vi "SECoP_dataGetInfo.vi"(7 "Position":u32, 8 "error in (no error)":errorcluster, 10 "SECoP_dataPtr":T1 {"ptr64" format="%.0x"; "ptr32" format="%.0x"}, 11 "DLL path (in)":T3) -> (0 "error out":errorcluster, 1 "Name":string, 2 "Type":T2 items=["NONE"=0, "DOUBLE"=1, "INTEGER"=2, "BOOL"=3, "ENUM"=4, "SCALED"=5, "ARRAY"=10, "ARRAY_DOUBLE"=11, "ARRAY_INTEGER"=12, "ARRAY_BOOL"=13, "ARRAY_ENUM"=14, "ARRAY_SCALED"=15, "STRING"=20, "BLOB"=21, "JSON"=22, "STRUCT"=30, "TUPLE"=31, "COMMAND"=40], 3 "DLL path (out)":T3, 5 "Count":u32)   [LabVIEW 2023, in "SECoP.lvlib"]
doc: "Call <b>\"SECoP_dataGetInfo.vi\"</b> to access the numeric value (integer or scaled of SECoP_dataPtr).\n\n<b>DLL path</b> input and output of cluster from \"SECoP-Initialize.vi\"\n<b>SECoP_dataPtr</b> data to access\n<b>Position</b> zero based index points to a virtual flattened entry of the data type\n<b>Type</b> data type of selected element\n<b>Count</b> for array/struct/tuple a length or count of elements, for single type should be 1\n<b>Name</b> name of selected structure item or empty (no struct)"
uses:
  SECoP.lvlib
  SECoP-libraries.ctl
  SECoP-dataType.ctl
  SECoP-data.ctl
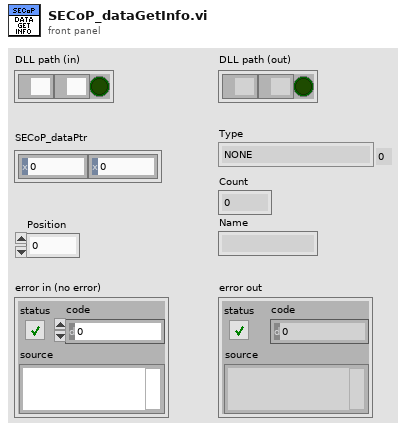
[diagram p1: front panel]
types:
  T1 = typedef "SECoP.lvlib/SECoP-data.ctl" = cluster{"ptr32":u32, "ptr64":u64}
  T2 = typedef "SECoP.lvlib/SECoP-dataType.ctl" = u32
  T3 = typedef "SECoP.lvlib/SECoP-libraries.ctl" = cluster{"serverDLL":path, "variantDLL":path, "cleanup_mode":bool}
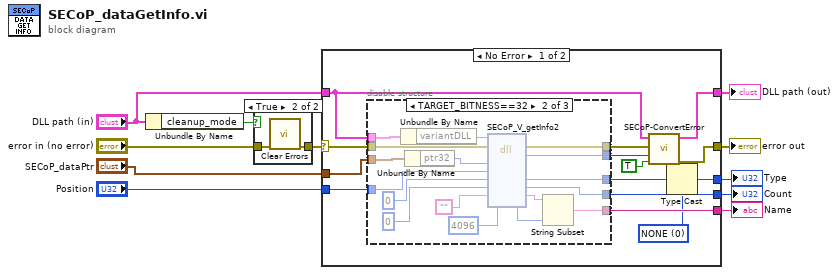
[diagram p0: block diagram]
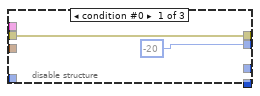
[diagram p3: hidden frame]
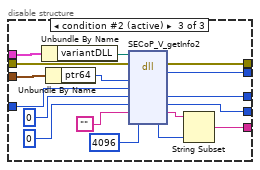
[diagram p4: hidden frame]
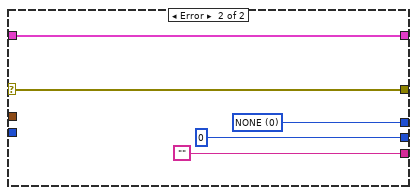
[diagram p5: hidden frame]
diagram:
  n1 = Unbundle By Name("DLL path (in)") -> ("cleanup_mode"=w8:bool)
  n2 = case shown="True" w8 {
    tunnel: "error in (no error)" -> [w12 w14]
    tunnel: [w12 w13] -> w6
    frame False {
    }
    frame True {
      n3 = call <vilib>:"Clear Errors.vi"("error in (no error)"=w14) -> ("error out"=w13:errorcluster)  [unwired: 5 in, 1 out]
    }
  }
  n4 = case shown="No Error" w6 {
    selector: w6 -> [w26 w68]
    tunnel: "DLL path (in)" -> [w18 w69]
    tunnel: [w27 w69] -> w10
    tunnel: [w28 w68] -> w9
    tunnel: "Position" -> [w23 _]
    tunnel: [w15 w65] -> w4
    tunnel: [w21 ""] -> w3
    tunnel: [w22 u32 0 ("Count")] -> w2
    tunnel: "SECoP_dataPtr" -> [w19 _]
    frame No Error {
      w16 = T2 0 items=["NONE"=0, "DOUBLE"=1, "INTEGER"=2, "BOOL"=3, "ENUM"=4, "SCALED"=5, "ARRAY"=10, "ARRAY_DOUBLE"=11, "ARRAY_INTEGER"=12, "ARRAY_BOOL"=13, "ARRAY_ENUM"=14, "ARRAY_SCALED"=15, "STRING"=20, "BLOB"=21, "JSON"=22, "STRUCT"=30, "TUPLE"=31, "COMMAND"=40] ("SECoP data type")
      n5 = disable-structure shown="TARGET_BITNESS==32" {
        disable-tunnel: w26 -> [w30 w47 w64]
        disable-tunnel: w18 -> [_ w46 w63]
        disable-tunnel: [w30 w45 w62] -> w25
        disable-tunnel: [-20 w44 w61] -> w24
        disable-tunnel: w23 -> [_ w43 w60]
        disable-tunnel: [_ w42 w59] -> w17
        disable-tunnel: [_ w40 w57] -> w22
        disable-tunnel: [_ w35 w52] -> w21
        disable-tunnel: w19 -> [_ w33 w51]
        frame condition #0 {
        }
        frame condition #1 {
          n6 = Unbundle By Name(w46) -> ("variantDLL"=w31:path)
          n7 = Unbundle By Name(w33) -> ("ptr32"=w32:u32)
          n8 = dll-call lib="Z:/Praktische_Aufgaben/SECoP-LabVIEW2015/32bit/SECoP32.dll" fn="SECoP_V_getInfo2"(path in=w31, error in=w47, "Data"=w32, "Position"=w43, "Type"=0, "Count"=u32 0, "Name"="", "name length"=4096) -> (error out=w45:errorcluster, "return type"=w44:i32, "Type"=w42:i32, "Count"=w40:u32, "Name"=w41:string, "name length"=w34:i32)  [unwired: 3 in, 1 out]
          n9 = String Subset(string=w41, length (rest)=w34) -> (substring=w35:string)  [unwired: 1 in]
        }
        frame condition #2 (active) {
          n10 = Unbundle By Name(w63) -> ("variantDLL"=w48:path)
          n11 = Unbundle By Name(w51) -> ("ptr64"=w50:u64)
          n12 = dll-call lib="Z:/Praktische_Aufgaben/SECoP-LabVIEW2015/32bit/SECoP32.dll" fn="SECoP_V_getInfo2"(path in=w48, error in=w64, "Data"=w50, "Position"=w60, "Type"=0, "Count"=u32 0, "Name"="", "name length"=4096) -> (error out=w62:errorcluster, "return type"=w61:i32, "Type"=w59:i32, "Count"=w57:u32, "Name"=w58:string, "name length"=w49:i32)  [unwired: 3 in, 1 out]
          n13 = String Subset(string=w58, length (rest)=w49) -> (substring=w52:string)  [unwired: 1 in]
        }
      }
      n14 = call "SECoP-ConvertError.vi"("return is boolean"=TRUE, "return code"=w24, "error in (no error)"=w25, "DLL path (in)"=w18) -> ("error out"=w28:errorcluster, "DLL path (out)"=w27:T3)  [unwired: 6 in]
      n15 = Type Cast(type=w16, x=w17) -> (*(type *) &x=w15:T2)
    }
    frame Error {
      w65 = T2 0 items=["NONE"=0, "DOUBLE"=1, "INTEGER"=2, "BOOL"=3, "ENUM"=4, "SCALED"=5, "ARRAY"=10, "ARRAY_DOUBLE"=11, "ARRAY_INTEGER"=12, "ARRAY_BOOL"=13, "ARRAY_ENUM"=14, "ARRAY_SCALED"=15, "STRING"=20, "BLOB"=21, "JSON"=22, "STRUCT"=30, "TUPLE"=31, "COMMAND"=40] ("SECoP data type")
    }
  }
  "DLL path (out)" <- w10
  "error out" <- w9
  "Type" <- w4
  "Count" <- w2
  "Name" <- w3
